vi "Write Label at Path.vi"   [LabVIEW 2020, in "Variant Data Manipulation.lvlib"]
uses:
  Variant Data Manipulation.lvlib
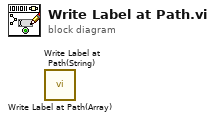
[diagram p0: block diagram]
diagram:
  n1 = call "Write Label at Path(Array).vi"() -> ()  [unwired: 10 in, 2 out]
  n2 = call "Write Label at Path(String).vi"() -> ()  [unwired: 10 in, 2 out]
